vi "GageSampInterval.vi"(3 "Sampling Rate":u16(ring)) -> (0 "Sampling Rate (MHz)":i32, 1 "time (s)":dbl format="%.2e")   [LabVIEW 2022 SP3]
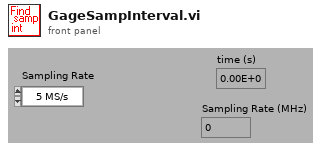
[diagram p1: front panel]
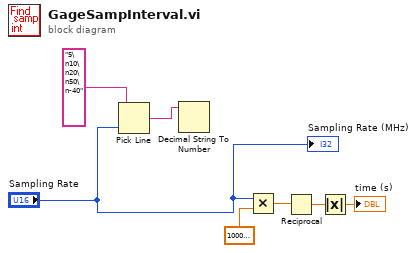
[diagram p0: block diagram]
diagram:
  n1 = Pick Line(multi-line string="5\n10\n20\n50\n-40", line index="Sampling Rate") -> (output string=w6:string)  [unwired: 1 out]
  n2 = Decimal String To Number(string=w6) -> ()  [unwired: 4 out]
  n3 = Multiply(x="Sampling Rate", y=1000000.0) -> (x*y=w4:dbl)
  n4 = Reciprocal(x=w4) -> (1/x=w3:dbl)
  n5 = Absolute Value(x=w3) -> (abs(x)=→"time (s)":dbl)
  "Sampling Rate (MHz)" <- "Sampling Rate"
